vi "play.vi"() -> ()   [LabVIEW 2014]
panel:
  out "Array 2":bool[][](array[boolean])
  out "Array":picture[][](array[picture])
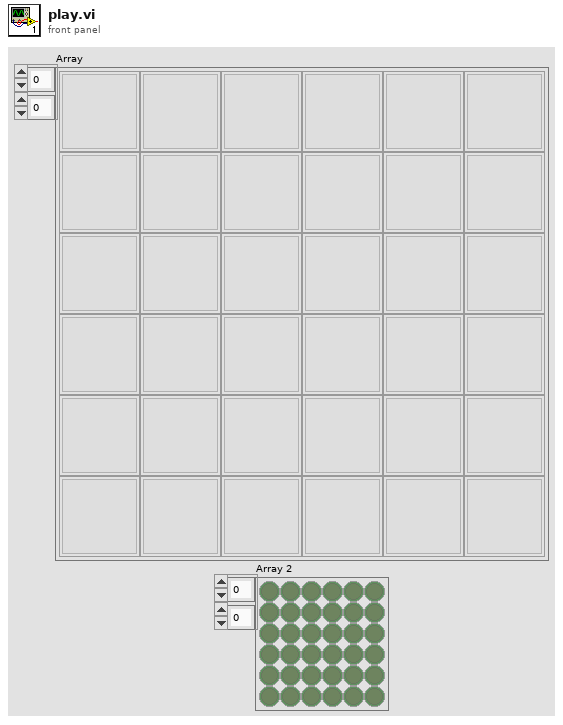
[diagram p1: front panel]
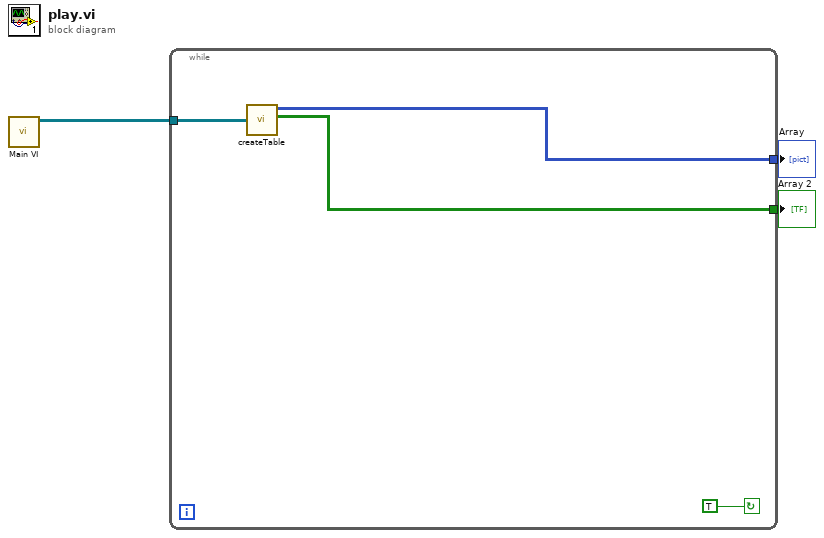
[diagram p0: block diagram]
diagram:
  n1 = call "Main VI.vi"() -> ("Output board"=w1:refnum<class "Cell.lvclass">[][])  [unwired: 11 in]
  n2 = while {
    tunnel: [w7] -> w3
    tunnel: [w5] -> w2
    tunnel: w1 -> [w4]
    stop <- TRUE continue-if-true
    n3 = call "createTable.vi"("Input board"=w4) -> ("Array 2"=w5:bool[][], "Array"=w7:picture[][])  [unwired: 9 in]
  }
  "Array" <- w3
  "Array 2" <- w2
